vi "Begin.vi"() -> (0 "error out":errorcluster)   [LabVIEW 2013]
doc: "Called before other user functions, this VI is expected to open initial I/O refnums, load in file data, and do all program initialization. Notice that the <B>error out</B> terminal is simply used for data flow. Wiring it to other structures or subVIs ensures that this VI runs first."
uses:
  <vilib>/Rock Robotics/WPI/Joystick/WPI_JoystickDeviceEnum.ctl
  <vilib>/Rock Robotics/SystemInterfaces/Typedef/FPGA_TypedefDigitalModule.ctl
  <vilib>/Rock Robotics/SystemInterfaces/DIO/FPGA_DIOChannel.ctl
  <vilib>/Rock Robotics/SystemInterfaces/DIO/FPGA_DIORelayChannel.ctl
  <vilib>/Rock Robotics/SystemInterfaces/Typedef/FPGA_TypedefSolenoidModule.ctl
  <vilib>/Rock Robotics/WPI/Solenoid/WPI_SolenoidChannel.ctl
  <vilib>/Rock Robotics/WPI/Solenoid/WPI_SolenoidValue.ctl
  <vilib>/Rock Robotics/SystemInterfaces/DIO/FPGA_DIOPWMChannel.ctl
  <vilib>/Rock Robotics/WPI/Encoder/WPI_EncoderType.ctl
  <vilib>/Rock Robotics/WPI/Solenoid/WPI_SolenoidOpenDouble.vi
  <vilib>/Rock Robotics/WPI/Solenoid/WPI_SolenoidSetEnum.vi
  <vilib>/Rock Robotics/WPI/Counter/WPI_CounterDigitalInputToDigitalSource.vi
  <vilib>/Rock Robotics/WPI/RobotDrive/WPI_RobotDriveOpen2MotorWithVictor.vi
  <vilib>/Rock Robotics/WPI/MotorControl/WPI_MotorControlOpen Jaguar.vi
  <vilib>/Rock Robotics/WPI/MotorControl/WPI_MotorControlOpen Victor.vi
  <vilib>/Rock Robotics/WPI/Compressor/WPI_CompressorGetSetRefNum.vi
  <vilib>/Rock Robotics/WPI/Camera/WPI_CameraImageSize.ctl
  <vilib>/Rock Robotics/WPI/Camera/WPI_CameraWhite Balance Values.ctl
  <vilib>/Rock Robotics/WPI/Camera/WPI_CameraExposure Values.ctl
  <vilib>/Rock Robotics/WPI/Camera/WPI_CameraFrameRate.ctl
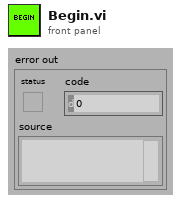
[diagram p1: front panel]
types:
  T1 = typedef "FPGA_DIOChannel.ctl" = enum8{"DIO 1", "DIO 2", "DIO 3", "DIO 4", "DIO 5", "DIO 6", "DIO 7", "DIO 8", "DIO 9", "DIO 10", "DIO 11", "DIO 12", "DIO 13", "DIO 14", "Invalid"}
  T2 = typedef "WPI_SolenoidValue.ctl" = enum16{"Off", "On", "Forward", "Reverse"}
  T3 = typedef "WPI_SolenoidChannel.ctl" = enum8{"Solenoid 1", "Solenoid 2", "Solenoid 3", "Solenoid 4", "Solenoid 5", "Solenoid 6", "Solenoid 7", "Solenoid 8", "Invalid"}
  T4 = typedef "FPGA_DIOPWMChannel.ctl" = enum8{"PWM 1", "PWM 2", "PWM 3", "PWM 4", "PWM 5", "PWM 6", "PWM 7", "PWM 8", "PWM 9", "PWM 10", "Invalid"}
  T5 = typedef "WPI_EncoderType.ctl" = enum16{"1x", "2x", "4x"}
  T6 = typedef "FPGA_TypedefSolenoidModule.ctl" = enum16{"Solenoid Module 1", "Solenoid Module 2"}
  T7 = typedef "FPGA_DIORelayChannel.ctl" = enum8{"Relay 1", "Relay 2", "Relay 3", "Relay 4", "Relay 5", "Relay 6", "Relay 7", "Relay 8", "Invalid"}
  T8 = typedef "WPI_JoystickDeviceEnum.ctl" = enum16{"USB 1", "USB 2", "USB 3", "USB 4", "Kinect 1", "Kinect 2"}
  T9 = typedef "FPGA_TypedefDigitalModule.ctl" = enum16{"Digital Module 1", "Digital Module 2"}
  T10 = typedef "WPI_CameraFrameRate.ctl" = u32
  T11 = typedef "WPI_CameraExposure Values.ctl" = enum16{"Auto", "Flicker-free 50 Hz", "Flicker-free 60 Hz", "Hold current"}
  T12 = typedef "WPI_CameraWhite Balance Values.ctl" = enum16{"Auto", "Fixed indoor", "Fixed outdoor 1", "Fixed outdoor 2", "Fixed fluorescent 1", "Fixed fluorescent 2", "Hold current"}
  T13 = typedef "WPI_CameraImageSize.ctl" = enum16{"640x480", "320x240", "160x120"}
  T14 = typedef "WPI_CameraDevRef.ctl" = cluster{"Camera Address":string, "CameraStatus":errorcluster, "Acquire Image Notifier":refnum<notifier>}
  T15 = typedef "WPI_DigitalInputDevRef.ctl" = cluster{"DevStatus":errorcluster, "DIO Channel":T1, "Digital Module":T9}
  T16 = typedef "WPI_MotorControlDeviceRef.ctl" = cluster{"DeviceStatus":errorcluster, "Type":enum16{"PWM", "CAN"}, "PWM":cluster{"Digital Module":T9, "PWM Channel":T4, "DeadBand":T17}, "CAN":cluster{"Device Number":u8, "Control Mode":T18, "Semaphore":T19, "Max Vout":dbl}, "Invert":bool, "TransformRef":T20, "InvTransformRef":T20}
  T17 = typedef "WPI_PWMDeadband.ctl" = cluster{"Name":string, "maxPositivePwm":i32, "minPositivePwm":i32, "centerPwm":i32, "maxNegativePwm":i32, "minNegativePwm":i32, "angularRange":u16}
  T18 = typedef "WPI_CANJaguar_ControlMode.ctl" = enum8{"Percent VBus", "Current", "Speed", "Position", "Voltage"}
  T19 = typedef "Semaphore RefNum" = refnum<k1>
  T20 = typedef "WPI_PWMTransform_ConPane.ctl" = refnum<vi>
  T21 = typedef "WPI_SolenoidDevRef.ctl" = cluster{"DevStatus":errorcluster, "Solenoid Module":T6, "Forward Solenoid Channel":T3, "Reverse Solenoid Channel":T3}
  T22 = typedef "FPGA_CounterEncoderSourceConvertionLVSourceType.ctl" = cluster{"DevStatus":errorcluster, "AnalogTriggerMode?":bool, "DigitalMode":cluster{"Digital Module":T9, "DIO Channel":T23}, "AnalogTriggerMode":cluster{"AnalogTriggerIndex":T24, "OutputType":T25}}
  T23 = typedef "FPGA_DIODigitalSourceChannel.ctl" = enum8{"DIO 1", "DIO 2", "DIO 3", "DIO 4", "DIO 5", "DIO 6", "DIO 7", "DIO 8", "DIO 9", "DIO 10", "DIO 11", "DIO 12", "DIO 13", "DIO 14", "Disabled"}
  T24 = typedef "FPGA_AnalogTriggerIndex.ctl" = enum8{"Trig 0", "Trig 1", "Trig 2", "Trig 3", "Trig 4", "Trig 5", "Trig 6", "Trig 7", "Invalid"}
  T25 = typedef "FPGA_AnalogTriggerOutType.ctl" = enum16{"InWindow", "TriggerState", "Rising", "Falling"}
  T26 = typedef "WPI_CompressorDevRef.ctl" = cluster{"DevStatus":errorcluster, "DigitalInputDevRef":T15, "RelayDevRef":T27}
  T27 = typedef "WPI_RelayDevRef.ctl" = cluster{"DevStatus":errorcluster, "Relay Channel":T7, "Digital Module":T9, "Relay Direction":T28}
  T28 = typedef "WPI_RelayDirection.ctl" = enum16{"Both directions", "Forward only", "Reverse only"}
  T29 = typedef "WPI_RobotDriveDevRef.ctl" = cluster{"DevStatus":errorcluster, "Motors[]":T16[], "Square Inputs":bool, "Max Output":dbl, "Isochronous":bool}
  T30 = typedef "WPI_EncoderDevRef.ctl" = cluster{"DevStatus":errorcluster, "EncoderIndex":T31, "CounterIndex":T32, "DistancePerCount":dbl, "Decoding Type":T5}
  T31 = typedef "FPGA_EncoderIdx.ctl" = enum8{"Enc 0", "Enc 1", "Enc 2", "Enc 3", "Invalid"}
  T32 = typedef "FPGA_CounterCtrSystemIndex.ctl" = enum8{"Ctr 0", "Ctr 1", "Ctr 2", "Ctr 3", "Ctr 4", "Ctr 5", "Ctr 6", "Ctr 7", "Invalid"}
  T33 = typedef "WPI_JoystickDevRef.ctl" = cluster{"Device":T8}
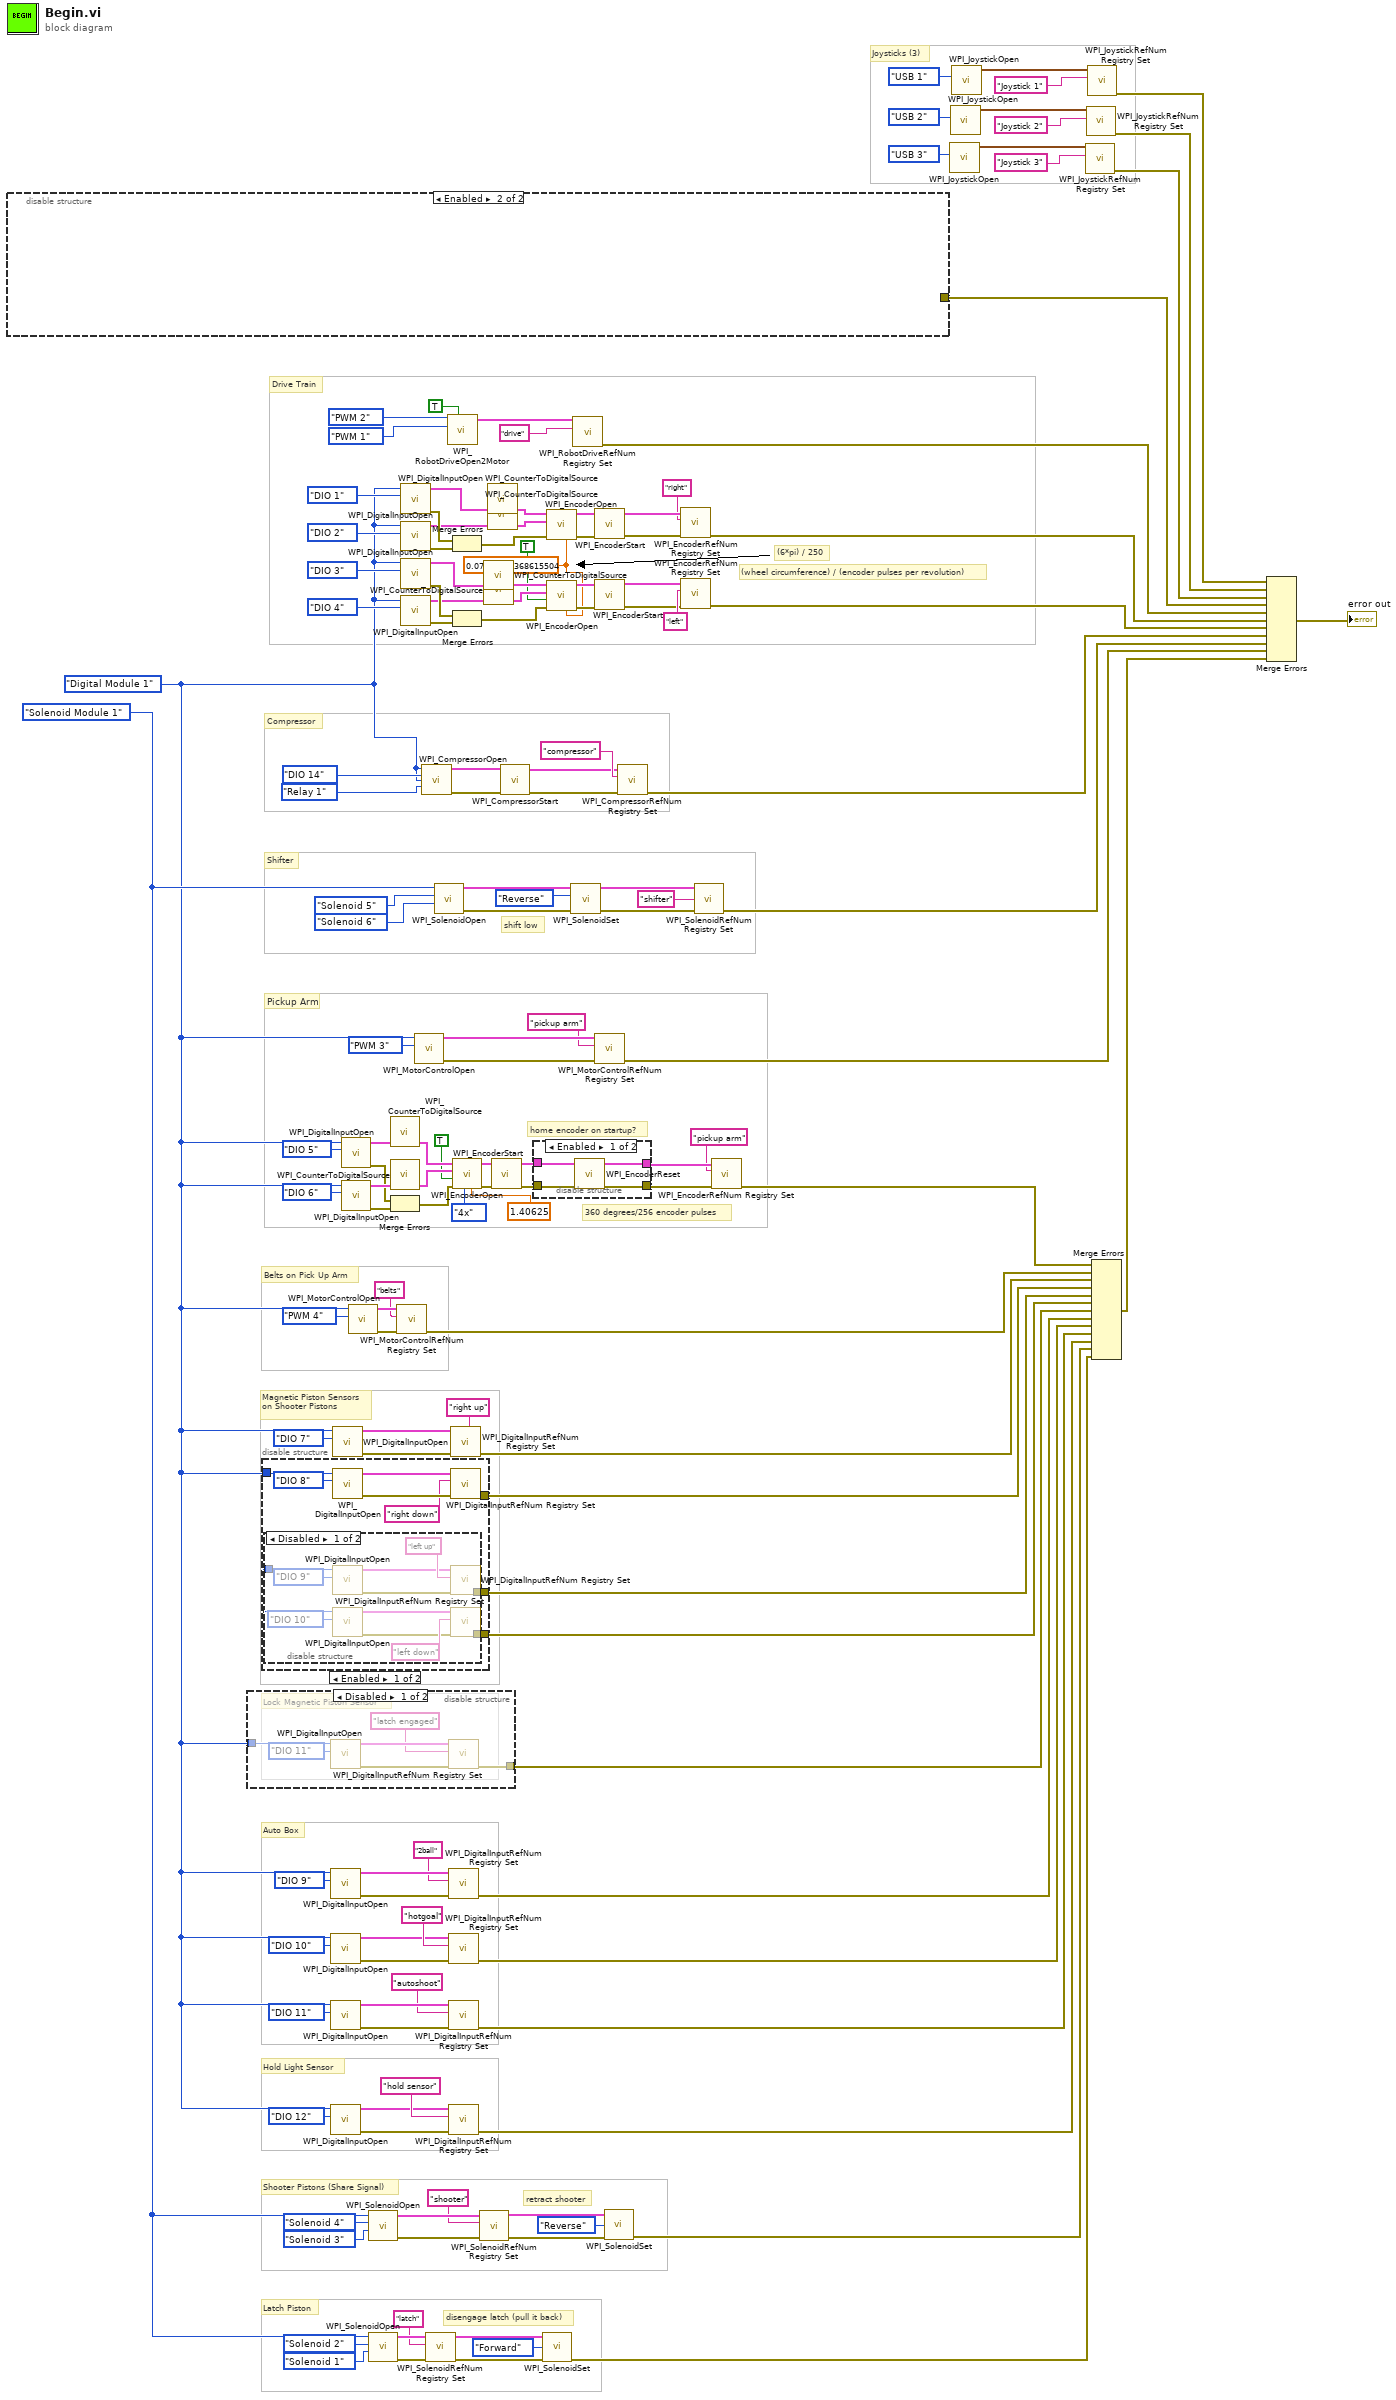
[diagram p0: block diagram]
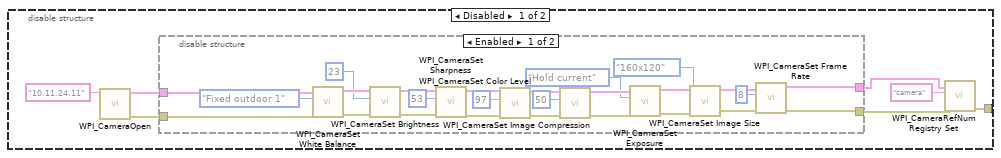
[diagram p2: hidden frame]
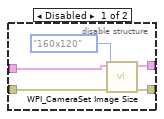
[diagram p4: hidden frame]
diagram:
  w93 = 0.07539822368615504 ("DistancePerCount")
  w36 = FPGA_TypedefSolenoidModule."Solenoid Module 1" ("Solenoid Module (Module 1)")
  w5 = FPGA_TypedefDigitalModule."Digital Module 1" ("Digital Module (Module 1)")
  # "Auto Box"
  # "retract shooter"
  # "disengage latch (pull it back)"
  # "360 degrees/256 encoder pulses"
  # "Hold Light Sensor"
  # "Joysticks (3)"
  # "Latch Piston"
  # "Shooter Pistons (Share Signal)"
  # "Magnetic Piston Sensors\non Shooter Pistons"
  # "Belts on Pick Up Arm"
  # "Pickup Arm"
  # "home encoder on startup?"
  # "Shifter"
  # "Compressor"
  # "Drive Train"
  # "shift low"
  # "(wheel circumference) / (encoder pulses per revolution)"
  # "(6*pi) / 250"
  n1 = disable-structure shown="Enabled" {
    disable-tunnel: [w156 _] -> w137
    frame Disabled {
      n2 = call <vilib>:"WPI_CameraOpen.vi"("Camera Address"="10.11.24.11") -> ("error out"=w151:errorcluster, "CameraDevRef"=w153:T14)  [unwired: 9 in]
      n3 = disable-structure shown="Enabled" {
        disable-tunnel: w153 -> [w180 w186]
        disable-tunnel: [w158 w185] -> w152
        disable-tunnel: w151 -> [w167 w184]
        disable-tunnel: [w157 w183] -> w150
        frame Enabled {
          n4 = call <vilib>:"WPI_CameraSet White Balance.vi"("error in (no error)"=w167, "White Balance"=WPI_CameraWhite_Balance_Values."Fixed outdoor 1", "CameraDevRef"=w180) -> ("error out"=w168:errorcluster, "CameraDevRef Out"=w179:T14)  [unwired: 7 in]
          n5 = call <vilib>:"WPI_CameraSet Brightness.vi"("error in (no error)"=w168, "Brightness"=23, "CameraDevRef"=w179) -> ("error out"=w169:errorcluster, "CameraDevRef Out"=w178:T14)  [unwired: 7 in]
          n6 = call <vilib>:"WPI_CameraSet Sharpness.vi"("error in (no error)"=w169, "Sharpness"=53, "CameraDevRef"=w178) -> ("error out"=w170:errorcluster, "CameraDevRef Out"=w177:T14)  [unwired: 7 in]
          n7 = call <vilib>:"WPI_CameraSet Color Level.vi"("error in (no error)"=w170, "Color Level"=97, "CameraDevRef"=w177) -> ("error out"=w171:errorcluster, "CameraDevRef Out"=w176:T14)  [unwired: 7 in]
          n8 = call <vilib>:"WPI_CameraSet Image Compression.vi"("error in (no error)"=w171, "Compression"=50, "CameraDevRef"=w176) -> ("error out"=w182:errorcluster, "CameraDevRef Out"=w181:T14)  [unwired: 7 in]
          n9 = call <vilib>:"WPI_CameraSet Exposure.vi"("error in (no error)"=w182, "Exposure"=WPI_CameraExposure_Values."Hold current", "CameraDevRef"=w181) -> ("error out"=w172:errorcluster, "CameraDevRef Out"=w175:T14)  [unwired: 7 in]
          n10 = call <vilib>:"WPI_CameraSet Image Size.vi"("error in (no error)"=w172, "Image Size"=WPI_CameraImageSize."160x120", "CameraDevRef"=w175) -> ("error out"=w173:errorcluster, "CameraDevRef Out"=w174:T14)  [unwired: 7 in]
          n11 = call <vilib>:"WPI_CameraSet Frame Rate.vi"("error in (no error)"=w173, "Frame Rate (fps)"=T10 8, "CameraDevRef"=w174) -> ("error out"=w157:errorcluster, "CameraDevRef Out"=w158:T14)  [unwired: 7 in]
        }
        frame Disabled {
          n12 = disable-structure shown="Enabled" {
            disable-tunnel: w184 -> [w190 w192]
            disable-tunnel: [w189 w192] -> w183
            disable-tunnel: w186 -> [w188 w193]
            disable-tunnel: [w187 w193] -> w185
            frame Disabled {
              n13 = call <vilib>:"WPI_CameraSet Image Size.vi"("error in (no error)"=w190, "Image Size"=WPI_CameraImageSize."160x120", "CameraDevRef"=w188) -> ("error out"=w189:errorcluster, "CameraDevRef Out"=w187:T14)  [unwired: 7 in]
            }
            frame Enabled {
            }
          }
        }
      }
      n14 = call <vilib>:"WPI_CameraRefNum Registry Set.vi"("error in (no error)"=w150, "refnum name"="camera", "CameraDevRef"=w152) -> ("error out"=w156:errorcluster)  [unwired: 7 in, 1 out]
    }
    frame Enabled {
    }
  }
  n15 = disable-structure shown="Disabled" {
    disable-tunnel: w5 -> [w195 _]
    disable-tunnel: [w194 _] -> w29
    frame Disabled {
      # "Lock Magnetic Piston Sensor"
      n16 = call <vilib>:"WPI_DigitalInputOpen.vi"("DIO Channel"=FPGA_DIOChannel."DIO 11", "Digital Module (Module 1)"=w195) -> ("error out"=w198:errorcluster, "DigitalInputDevRef"=w197:T15)  [unwired: 8 in]
      n17 = call <vilib>:"WPI_DigitalInputRefNum Registry Set.vi"("error in (no error)"=w198, "refnum name"="latch engaged", "DigitalInputDevRef"=w197) -> ("error out"=w194:errorcluster)  [unwired: 7 in, 1 out]
    }
    frame Enabled {
      # "no latch magnetic sensor"
    }
  }
  n18 = disable-structure shown="Enabled" {
    disable-tunnel: [w204 _] -> w47
    disable-tunnel: w5 -> [w202 _]
    disable-tunnel: [w201 _] -> w31
    disable-tunnel: [w200 _] -> w30
    frame Enabled {
      n19 = disable-structure shown="Disabled" {
        disable-tunnel: w202 -> [w210 _]
        disable-tunnel: [w209 _] -> w201
        disable-tunnel: [w208 _] -> w200
        frame Disabled {
          n20 = call <vilib>:"WPI_DigitalInputOpen.vi"("DIO Channel"=FPGA_DIOChannel."DIO 9", "Digital Module (Module 1)"=w210) -> ("error out"=w211:errorcluster, "DigitalInputDevRef"=w212:T15)  [unwired: 8 in]
          n21 = call <vilib>:"WPI_DigitalInputOpen.vi"("DIO Channel"=FPGA_DIOChannel."DIO 10", "Digital Module (Module 1)"=w210) -> ("error out"=w213:errorcluster, "DigitalInputDevRef"=w214:T15)  [unwired: 8 in]
          n22 = call <vilib>:"WPI_DigitalInputRefNum Registry Set.vi"("error in (no error)"=w211, "refnum name"="left up", "DigitalInputDevRef"=w212) -> ("error out"=w209:errorcluster)  [unwired: 7 in, 1 out]
          n23 = call <vilib>:"WPI_DigitalInputRefNum Registry Set.vi"("error in (no error)"=w213, "refnum name"="left down", "DigitalInputDevRef"=w214) -> ("error out"=w208:errorcluster)  [unwired: 7 in, 1 out]
        }
        frame Enabled {
        }
      }
      n24 = call <vilib>:"WPI_DigitalInputOpen.vi"("DIO Channel"=FPGA_DIOChannel."DIO 8", "Digital Module (Module 1)"=w202) -> ("error out"=w207:errorcluster, "DigitalInputDevRef"=w206:T15)  [unwired: 8 in]
      n25 = call <vilib>:"WPI_DigitalInputRefNum Registry Set.vi"("error in (no error)"=w207, "refnum name"="right down", "DigitalInputDevRef"=w206) -> ("error out"=w204:errorcluster)  [unwired: 7 in, 1 out]
    }
    frame Disabled {
      # "dang, only one sensor\non the pistons..."
    }
  }
  n26 = call <vilib>:"WPI_DigitalInputOpen.vi"("DIO Channel"=FPGA_DIOChannel."DIO 9", "Digital Module (Module 1)"=w5) -> ("error out"=w17:errorcluster, "DigitalInputDevRef"=w16:T15)  [unwired: 8 in]
  n27 = call <vilib>:"WPI_DigitalInputOpen.vi"("DIO Channel"=FPGA_DIOChannel."DIO 10", "Digital Module (Module 1)"=w5) -> ("error out"=w12:errorcluster, "DigitalInputDevRef"=w13:T15)  [unwired: 8 in]
  n28 = call <vilib>:"WPI_DigitalInputOpen.vi"("DIO Channel"=FPGA_DIOChannel."DIO 11", "Digital Module (Module 1)"=w5) -> ("error out"=w8:errorcluster, "DigitalInputDevRef"=w7:T15)  [unwired: 8 in]
  n29 = call <vilib>:"WPI_DigitalInputOpen.vi"("DIO Channel"=FPGA_DIOChannel."DIO 12", "Digital Module (Module 1)"=w5) -> ("error out"=w33:errorcluster, "DigitalInputDevRef"=w34:T15)  [unwired: 8 in]
  n30 = call <vilib>:"WPI_DigitalInputOpen.vi"("DIO Channel"=FPGA_DIOChannel."DIO 7", "Digital Module (Module 1)"=w5) -> ("error out"=w52:errorcluster, "DigitalInputDevRef"=w51:T15)  [unwired: 8 in]
  n31 = call <vilib>:"WPI_DigitalInputOpen.vi"("DIO Channel"=FPGA_DIOChannel."DIO 5", "Digital Module (Module 1)"=w5) -> ("error out"=w69:errorcluster, "DigitalInputDevRef"=w74:T15)  [unwired: 8 in]
  n32 = call <vilib>:"WPI_DigitalInputOpen.vi"("DIO Channel"=FPGA_DIOChannel."DIO 6", "Digital Module (Module 1)"=w5) -> ("error out"=w70:errorcluster, "DigitalInputDevRef"=w73:T15)  [unwired: 8 in]
  n33 = call-poly <vilib>:"WPI_MotorControlOpen.vi"("PWM Channel"=FPGA_DIOPWMChannel."PWM 4", "Digital Module (Module 1)"=w5) -> ("error out"=w58:errorcluster, "MotorControlDeviceRef"=w57:T16)  [unwired: 8 in]
  n34 = call-poly <vilib>:"WPI_SolenoidOpen.vi"("Reverse Solenoid Channel"=WPI_SolenoidChannel."Solenoid 3", "Forward Solenoid Channel"=WPI_SolenoidChannel."Solenoid 4", "Solenoid Module (Module 1)"=w36) -> ("error out"=w42:errorcluster, "SolenoidDevRef"=w41:T21)  [unwired: 7 in]
  n35 = call-poly <vilib>:"WPI_SolenoidOpen.vi"("Reverse Solenoid Channel"=WPI_SolenoidChannel."Solenoid 1", "Forward Solenoid Channel"=WPI_SolenoidChannel."Solenoid 2", "Solenoid Module (Module 1)"=w36) -> ("error out"=w40:errorcluster, "SolenoidDevRef"=w39:T21)  [unwired: 7 in]
  n36 = call-poly <vilib>:"WPI_CounterToDigitalSource.vi"("DigitalInputDevRef"=w74) -> ("Digital Source"=w72:T22)  [unwired: 6 in]
  n37 = call-poly <vilib>:"WPI_CounterToDigitalSource.vi"("DigitalInputDevRef"=w73) -> ("Digital Source"=w71:T22)  [unwired: 6 in]
  n38 = Merge Errors(w69, w70) -> (w68:errorcluster)
  n39 = call <vilib>:"WPI_MotorControlRefNum Registry Set.vi"("error in (no error)"=w58, "refnum name"="belts", "MotorControlDevRef"=w57) -> ("error out"=w55:errorcluster)  [unwired: 7 in, 1 out]
  n40 = call <vilib>:"WPI_DigitalInputOpen.vi"("DIO Channel"=FPGA_DIOChannel."DIO 1", "Digital Module (Module 1)"=w5) -> ("error out"=w87:errorcluster, "DigitalInputDevRef"=w101:T15)  [unwired: 8 in]
  n41 = call <vilib>:"WPI_DigitalInputOpen.vi"("DIO Channel"=FPGA_DIOChannel."DIO 2", "Digital Module (Module 1)"=w5) -> ("error out"=w89:errorcluster, "DigitalInputDevRef"=w86:T15)  [unwired: 8 in]
  n42 = call <vilib>:"WPI_DigitalInputOpen.vi"("DIO Channel"=FPGA_DIOChannel."DIO 3", "Digital Module (Module 1)"=w5) -> ("error out"=w90:errorcluster, "DigitalInputDevRef"=w115:T15)  [unwired: 8 in]
  n43 = call <vilib>:"WPI_DigitalInputOpen.vi"("DIO Channel"=FPGA_DIOChannel."DIO 4", "Digital Module (Module 1)"=w5) -> ("error out"=w92:errorcluster, "DigitalInputDevRef"=w85:T15)  [unwired: 8 in]
  n44 = call-poly <vilib>:"WPI_MotorControlOpen.vi"("PWM Channel"=FPGA_DIOPWMChannel."PWM 3", "Digital Module (Module 1)"=w5) -> ("error out"=w81:errorcluster, "MotorControlDeviceRef"=w80:T16)  [unwired: 8 in]
  n45 = call <vilib>:"WPI_CompressorOpen.vi"("Pressure Switch Digital Module (Module 1)"=w5, "Pressure Switch DIO Channel"=FPGA_DIOChannel."DIO 14", "Relay Digital Module (Module 1)"=w5, "Relay Channel"=FPGA_DIORelayChannel."Relay 1") -> ("CompressorDevRef"=w129:T26, "error out"=w128:errorcluster)  [unwired: 10 in]
  n46 = call <vilib>:"WPI_SolenoidRefNum Registry Set.vi"("error in (no error)"=w40, "refnum name"="latch", "SolenoidDevRef"=w39) -> ("error out"=w27:errorcluster, "SolenoidDevRef"=w26:T21)  [unwired: 7 in]
  n47 = call-poly <vilib>:"WPI_SolenoidOpen.vi"("Reverse Solenoid Channel"=WPI_SolenoidChannel."Solenoid 6", "Forward Solenoid Channel"=WPI_SolenoidChannel."Solenoid 5", "Solenoid Module (Module 1)"=w36) -> ("error out"=w120:errorcluster, "SolenoidDevRef"=w121:T21)  [unwired: 7 in]
  n48 = call-poly <vilib>:"WPI_RobotDriveOpen2Motor.vi"("Left Motor Inverted"=TRUE, "Right Motor"=FPGA_DIOPWMChannel."PWM 1", "Left Motor"=FPGA_DIOPWMChannel."PWM 2") -> ("RobotDriveDevRef"=w117:T29)  [unwired: 7 in, 1 out]
  n49 = call <vilib>:"WPI_DigitalInputRefNum Registry Set.vi"("error in (no error)"=w17, "refnum name"="2ball", "DigitalInputDevRef"=w16) -> ("error out"=w25:errorcluster)  [unwired: 7 in, 1 out]
  n50 = call <vilib>:"WPI_DigitalInputRefNum Registry Set.vi"("error in (no error)"=w12, "refnum name"="hotgoal", "DigitalInputDevRef"=w13) -> ("error out"=w10:errorcluster)  [unwired: 7 in, 1 out]
  n51 = call <vilib>:"WPI_DigitalInputRefNum Registry Set.vi"("error in (no error)"=w8, "refnum name"="autoshoot", "DigitalInputDevRef"=w7) -> ("error out"=w1:errorcluster)  [unwired: 7 in, 1 out]
  n52 = call <vilib>:"WPI_DigitalInputRefNum Registry Set.vi"("error in (no error)"=w33, "refnum name"="hold sensor", "DigitalInputDevRef"=w34) -> ("error out"=w2:errorcluster)  [unwired: 7 in, 1 out]
  n53 = call <vilib>:"WPI_DigitalInputRefNum Registry Set.vi"("error in (no error)"=w52, "refnum name"="right up", "DigitalInputDevRef"=w51) -> ("error out"=w48:errorcluster)  [unwired: 7 in, 1 out]
  n54 = Merge Errors(w87, w89) -> (w88:errorcluster)
  n55 = Merge Errors(w90, w92) -> (w91:errorcluster)
  n56 = call <vilib>:"WPI_EncoderOpen.vi"("DistancePerCount"=1.40625, "Decoding Type"=WPI_EncoderType."4x", "error in (no error)"=w68, "Invert Direction (False)"=TRUE, "BSource"=w71, "ASource"=w72) -> ("error out"=w67:errorcluster, "EncoderDevRef"=w66:T30)  [unwired: 4 in]
  n57 = call <vilib>:"WPI_SolenoidRefNum Registry Set.vi"("error in (no error)"=w42, "refnum name"="shooter", "SolenoidDevRef"=w41) -> ("error out"=w21:errorcluster, "SolenoidDevRef"=w22:T21)  [unwired: 7 in]
  n58 = call-poly <vilib>:"WPI_CounterToDigitalSource.vi"("DigitalInputDevRef"=w115) -> ("Digital Source"=w108:T22)  [unwired: 6 in]
  n59 = call-poly <vilib>:"WPI_CounterToDigitalSource.vi"("DigitalInputDevRef"=w85) -> ("Digital Source"=w109:T22)  [unwired: 6 in]
  n60 = call-poly <vilib>:"WPI_CounterToDigitalSource.vi"("DigitalInputDevRef"=w101) -> ("Digital Source"=w107:T22)  [unwired: 6 in]
  n61 = call-poly <vilib>:"WPI_CounterToDigitalSource.vi"("DigitalInputDevRef"=w86) -> ("Digital Source"=w106:T22)  [unwired: 6 in]
  n62 = call <vilib>:"WPI_EncoderStart.vi"("error in (no error)"=w67, "EncoderDevRef"=w66) -> ("error out"=w65:errorcluster, "EncoderDevRef"=w64:T30)  [unwired: 8 in]
  n63 = call <vilib>:"WPI_CompressorStart.vi"("error in (no error)"=w128, "CompressorDevRef"=w129) -> ("error out"=w127:errorcluster, "CompressorDevRef"=w126:T26)  [unwired: 8 in]
  n64 = disable-structure shown="Enabled" {
    disable-tunnel: w65 -> [w222 w223]
    disable-tunnel: w64 -> [w221 w224]
    disable-tunnel: [w220 w224] -> w62
    disable-tunnel: [w219 w223] -> w63
    frame Enabled {
      n65 = call <vilib>:"WPI_EncoderReset.vi"("error in (no error)"=w222, "EncoderDevRef"=w221) -> ("error out"=w219:errorcluster, "EncoderDevRef"=w220:T30)  [unwired: 8 in]
    }
    frame Disabled {
    }
  }
  n66 = call-poly <vilib>:"WPI_SolenoidSet.vi"("error in (no error)"=w27, "Value"=WPI_SolenoidValue."Forward", "SolenoidDevRef"=w26) -> ("error out"=w4:errorcluster)  [unwired: 7 in, 1 out]
  n67 = call <vilib>:"WPI_EncoderOpen.vi"("DistancePerCount"=w93, "error in (no error)"=w88, "BSource"=w106, "ASource"=w107) -> ("error out"=w105:errorcluster, "EncoderDevRef"=w104:T30)  [unwired: 6 in]
  n68 = call <vilib>:"WPI_EncoderOpen.vi"("DistancePerCount"=w93, "error in (no error)"=w91, "Invert Direction (False)"=TRUE, "BSource"=w109, "ASource"=w108) -> ("error out"=w110:errorcluster, "EncoderDevRef"=w111:T30)  [unwired: 5 in]
  n69 = call-poly <vilib>:"WPI_SolenoidSet.vi"("error in (no error)"=w120, "Value"=WPI_SolenoidValue."Reverse", "SolenoidDevRef"=w121) -> ("error out"=w119:errorcluster, "SolenoidDevRef"=w118:T21)  [unwired: 7 in]
  n70 = call <vilib>:"WPI_RobotDriveRefNum Registry Set.vi"("refnum name"="drive", "RobotDriveDevRef"=w117) -> ("error out"=w136:errorcluster)  [unwired: 8 in, 1 out]
  n71 = call <vilib>:"WPI_EncoderStart.vi"("error in (no error)"=w105, "EncoderDevRef"=w104) -> ("error out"=w103:errorcluster, "EncoderDevRef"=w102:T30)  [unwired: 8 in]
  n72 = call <vilib>:"WPI_EncoderStart.vi"("error in (no error)"=w110, "EncoderDevRef"=w111) -> ("error out"=w112:errorcluster, "EncoderDevRef"=w113:T30)  [unwired: 8 in]
  n73 = call <vilib>:"WPI_MotorControlRefNum Registry Set.vi"("error in (no error)"=w81, "refnum name"="pickup arm", "MotorControlDevRef"=w80) -> ("error out"=w77:errorcluster)  [unwired: 7 in, 1 out]
  n74 = call-poly <vilib>:"WPI_SolenoidSet.vi"("error in (no error)"=w21, "Value"=WPI_SolenoidValue."Reverse", "SolenoidDevRef"=w22) -> ("error out"=w3:errorcluster)  [unwired: 7 in, 1 out]
  n75 = call <vilib>:"WPI_CompressorRefNum Registry Set.vi"("error in (no error)"=w127, "refnum name"="compressor", "CompressorDevRef"=w126) -> ("error out"=w82:errorcluster)  [unwired: 7 in, 1 out]
  n76 = call <vilib>:"WPI_EncoderRefNum Registry Set.vi"("error in (no error)"=w103, "refnum name"="right", "EncoderDevRef"=w102) -> ("error out"=w135:errorcluster)  [unwired: 7 in, 1 out]
  n77 = call <vilib>:"WPI_EncoderRefNum Registry Set.vi"("error in (no error)"=w112, "refnum name"="left", "EncoderDevRef"=w113) -> ("error out"=w134:errorcluster)  [unwired: 7 in, 1 out]
  n78 = call <vilib>:"WPI_SolenoidRefNum Registry Set.vi"("error in (no error)"=w119, "refnum name"="shifter", "SolenoidDevRef"=w118) -> ("error out"=w83:errorcluster)  [unwired: 7 in, 1 out]
  n79 = call <vilib>:"WPI_EncoderRefNum Registry Set.vi"("error in (no error)"=w63, "refnum name"="pickup arm", "EncoderDevRef"=w62) -> ("error out"=w54:errorcluster)  [unwired: 7 in, 1 out]
  n80 = call <vilib>:"WPI_JoystickOpen.vi"("JoystickDevice"=WPI_JoystickDeviceEnum."USB 3") -> ("JoystickDevRef"=w148:T33)  [unwired: 10 in]
  n81 = call <vilib>:"WPI_JoystickOpen.vi"("JoystickDevice"=WPI_JoystickDeviceEnum."USB 2") -> ("JoystickDevRef"=w145:T33)  [unwired: 10 in]
  n82 = call <vilib>:"WPI_JoystickOpen.vi"("JoystickDevice"=WPI_JoystickDeviceEnum."USB 1") -> ("JoystickDevRef"=w142:T33)  [unwired: 10 in]
  n83 = call <vilib>:"WPI_JoystickRefNum Registry Set.vi"("refnum name"="Joystick 3", "JoystickDevRef"=w148) -> ("error out"=w138:errorcluster)  [unwired: 8 in, 1 out]
  n84 = call <vilib>:"WPI_JoystickRefNum Registry Set.vi"("refnum name"="Joystick 2", "JoystickDevRef"=w145) -> ("error out"=w139:errorcluster)  [unwired: 8 in, 1 out]
  n85 = call <vilib>:"WPI_JoystickRefNum Registry Set.vi"("refnum name"="Joystick 1", "JoystickDevRef"=w142) -> ("error out"=w140:errorcluster)  [unwired: 8 in, 1 out]
  n86 = Merge Errors(w54, w55, w48, w47, w31, w30, w29, w25, w10, w1, w2, w3, w4) -> (w53:errorcluster)
  n87 = Merge Errors(w140, w139, w138, w137, w136, w135, w134, w82, w83, w77, w53) -> (→"error out":errorcluster)
